vi "Cleanup Session.vi"(8 "error in":errorcluster, 11 "Plugin in":refnum<class "Sift Stream.lvclass">) -> (0 "error out":errorcluster, 3 "Plugin out":refnum<class "Sift Stream.lvclass">)   [LabVIEW 2024, in "Sift Stream.lvlib" / "Sift Stream.lvclass"]
uses:
  Sift Stream.lvclass
  Sift Stream.lvclass/Sift Stream.ctl
  <vilib>/Sift/Sift/Sift API/Sift Client.lvclass
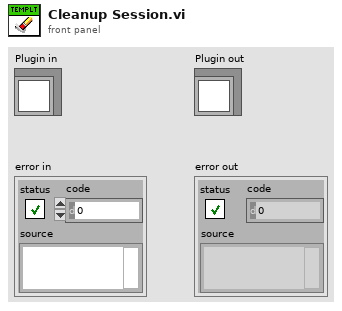
[diagram p1: front panel]
types:
  T1 = typedef "Sift Stream.lvlib/Sift Stream.lvclass/Sift Stream Parameters.ctl" = cluster{"API gRPC URL":string, "API REST URL":string, "API Key":string, "Asset Name":string, "Data Rate":dbl, "Stream Names":string[], "Buffer Size":i32, "Sift Client":refnum<class "Sift Client.lvclass">}
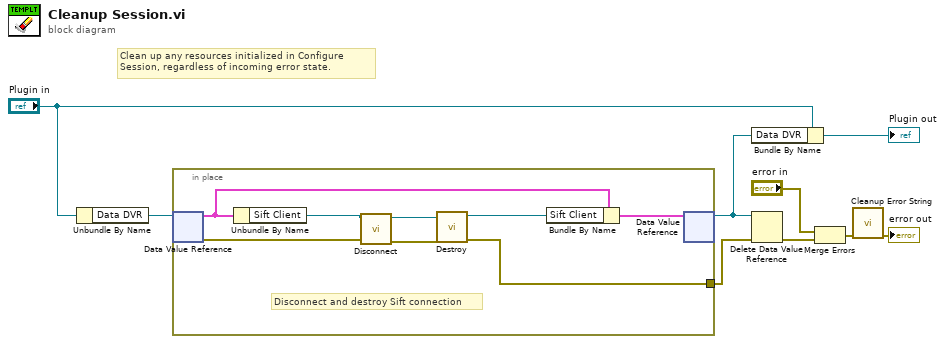
[diagram p0: block diagram]
diagram:
  # "Clean up any resources initialized in Configure Session, regardless of incoming error state."
  n1 = Unbundle By Name("Plugin in") -> ("Data DVR"=w9:refnum<data-value>)
  n2 = in-place {
    in-place-border: [w10] -> w7
    # "Disconnect and destroy Sift connection"
    n3 = in-place-dvr #1(w9) -> (w12:T1, w15:errorcluster)
    n4 = Unbundle By Name(w12) -> ("Sift Client"=w17:refnum<class "Sift Client.lvclass">)
    n5 = call-dynamic "Disconnect.vi"("error in (no error)"=w15, "Sift Client in"=w17) -> ("error out"=w14:errorcluster, "Sift Client out"=w16:refnum<class "Sift Client.lvclass">)  [unwired: 8 in]
    n6 = call-dynamic "Destroy.vi"("error in (no error)"=w14, "Sift Client in"=w16) -> ("error out"=w10:errorcluster, "Sift Client out"=w11:refnum<class "Sift Client.lvclass">)  [unwired: 8 in]
    n7 = Bundle By Name(cluster=w12, "Sift Client"=w11) -> (w13:T1)
    n8 = in-place-dvr #1(w13) -> (w8:refnum<data-value>)  [unwired: 1 out]
  }
  n9 = Bundle By Name(cluster="Plugin in", "Data DVR"=w8) -> (→"Plugin out":refnum<class "Sift Stream.lvclass">)
  n10 = Delete Data Value Reference(data value reference=w8, error in=w7) -> (error out=w6:errorcluster)  [unwired: 1 out]
  n11 = Merge Errors("error in", w6) -> (w2:errorcluster)
  n12 = call "Cleanup Error String.vi"("error in (no error)"=w2) -> ("error out"=→"error out":errorcluster)  [unwired: 10 in]
